vi "HiFiveUnmatched_MakeChannelCfg.vi"(9 "Power Line Identifier":T2, 10 "Enable":bool, 11 "Physical Channel":tag) -> (3 "Configuration":T1={"Name"="", "Shunt [Ohm]"=0.0, "Min Current [A]"=0.0, "Max Current [A]"=0.0, "Voltage [V]"=0.0, "Physical Channel"="", "Enable"=TRUE})   [LabVIEW 2020]
uses:
  HiFiveUnmatched_PowerLineId.ctl
  HiFiveUnmatched_PowerLineCfg.ctl
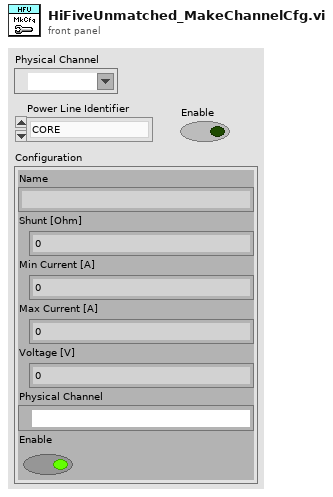
[diagram p1: front panel]
types:
  T1 = typedef "HiFiveUnmatched_PowerLineCfg.ctl" = cluster{"Name":string, "Shunt [Ohm]":dbl, "Min Current [A]":dbl, "Max Current [A]":dbl, "Voltage [V]":dbl, "Physical Channel":tag, "Enable":bool}
  T2 = typedef "HiFiveUnmatched_PowerLineId.ctl" = enum8{"CORE", "DDR_SOC", "IO", "PLL", "PCIEVP", "PCIEVPH", "DDR_MEM", "DDR_PLL", "DDR_VPP"}
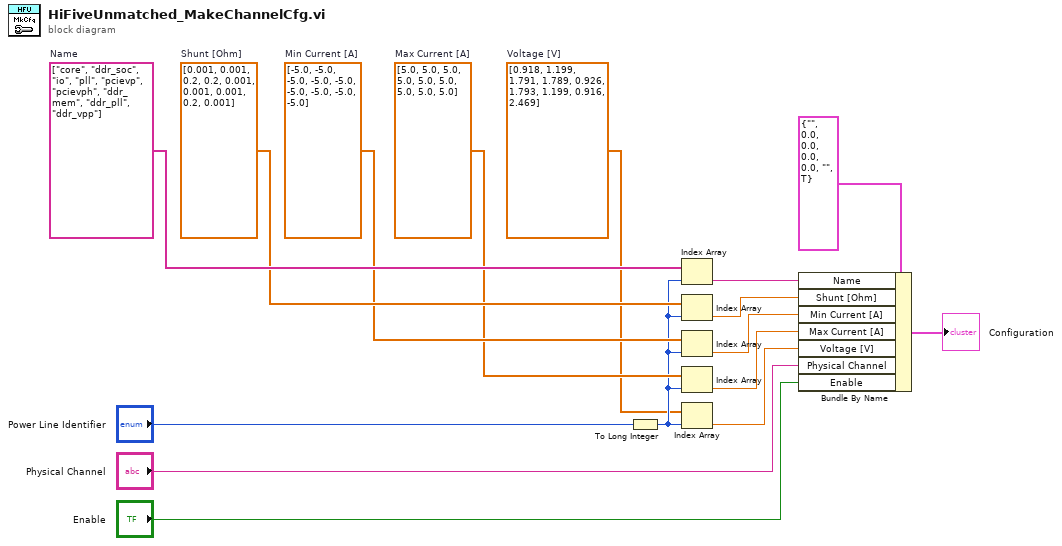
[diagram p0: block diagram]
diagram:
  w5 = dbl[] [0.918, 1.199, 1.791, 1.789, 0.926, 1.793, 1.199, 0.916, 2.469]  # Voltage [V]
  w13 = dbl[] [5.0, 5.0, 5.0, 5.0, 5.0, 5.0, 5.0, 5.0, 5.0]  # Max Current [A]
  w14 = dbl[] [-5.0, -5.0, -5.0, -5.0, -5.0, -5.0, -5.0, -5.0, -5.0]  # Min Current [A]
  w15 = dbl[] [0.001, 0.001, 0.2, 0.2, 0.001, 0.001, 0.001, 0.2, 0.001]  # Shunt [Ohm]
  w16 = string[] ["core", "ddr_soc", "io", "pll", "pcievp", "pcievph", "ddr_mem", "ddr_pll", "ddr_vpp"]  # Name
  n1 = To Long Integer(number="Power Line Identifier") -> (32bit integer=w6:i32)
  n2 = Index Array(array=w16, index=w6) -> (element=w10:string)
  n3 = Index Array(array=w15, index=w6) -> (element=w9:dbl)
  n4 = Index Array(array=w14, index=w6) -> (element=w8:dbl)
  n5 = Index Array(array=w13, index=w6) -> (element=w7:dbl)
  n6 = Index Array(array=w5, index=w6) -> (element=w4:dbl)
  n7 = Bundle By Name(cluster=T1 {"Name"="", "Shunt [Ohm]"=0.0, "Min Current [A]"=0.0, "Max Current [A]"=0.0, "Voltage [V]"=0.0, "Physical Channel"="", "Enable"=TRUE} ("HiFiveUnmatched_PowerLineCfg"), "Name"=w10, "Shunt [Ohm]"=w9, "Min Current [A]"=w8, "Max Current [A]"=w7, "Voltage [V]"=w4, "Physical Channel"="Physical Channel", "Enable"="Enable") -> (→"Configuration":T1)
